vi "InitAppData.vi"(8 "error in (no error)":errorcluster, 10 "Measurement Directory":path) -> (0 "error out":errorcluster, 3 "Application Data":T1)   [LabVIEW 2019]
uses:
  Typedefs/#cluster_ApplicationData.ctl
  <vilib>/ActorFramework/Message Enqueuer/Message Enqueuer.lvclass
  Typedefs/Acquisition Thread/#cluster_AcqQueueData.ctl
  Typedefs/Acquisition Thread/#enum_AcquisitionTask.ctl
  Typedefs/Saving Thread/#cluster_SavingQueueData.ctl
  Typedefs/Saving Thread/#enum_SavingTask.ctl
  ViewerManager/ViewerManager/ViewerManager.lvclass
  C:/Program Files (x86)/National Instruments/LabVIEW 2019/vi.lib/ActorFramework/Actor/Actor.lvclass
  ViewerManager/ViewerManager Messages/UpdateMeasurementDirectory Msg/UpdateMeasurementDirectory Msg.lvclass/UpdateMeasurementDirectory Msg.ctl
  <vilib>/ActorFramework/Message Enqueuer/Message Enqueuer.lvclass/Message Enqueuer.ctl
  <vilib>/ActorFramework/Message Enqueuer/Enqueue.vi
  ViewerManager/ViewerManager Messages/UpdateMeasurementDirectory Msg/UpdateMeasurementDirectory Msg.lvclass
  C:/Program Files (x86)/National Instruments/LabVIEW 2019/vi.lib/ActorFramework/Message/Message.lvclass
  <vilib>/Utility/LVClass/Get LV Class Name.vi
  <resource>/AFDebug/Generate Trace for Message.vi
  <vilib>/ActorFramework/Message Priority Queue/Priority Enqueue.vi
  <vilib>/ActorFramework/Actor/Actor.lvclass
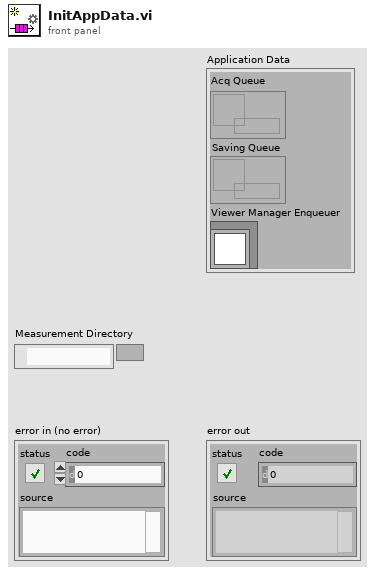
[diagram p1: front panel]
types:
  T1 = typedef "#cluster_ApplicationData.ctl" = cluster{"Acq Queue":refnum<queue>, "Saving Queue":refnum<queue>, "Viewer Manager Enqueuer":refnum<class "Message Enqueuer.lvclass">}
  T2 = typedef "#cluster_SavingQueueData.ctl" = cluster{"Task":T3, "Data":variant}
  T3 = typedef "#enum_SavingTask.ctl" = enum16{"Set directory", "Save", "Stop", "Close"}
  T4 = typedef "#cluster_AcqQueueData.ctl" = cluster{"Task":T5, "Data":variant}
  T5 = typedef "#enum_AcquisitionTask.ctl" = enum16{"Init", "Start", "Finish", "Close"}
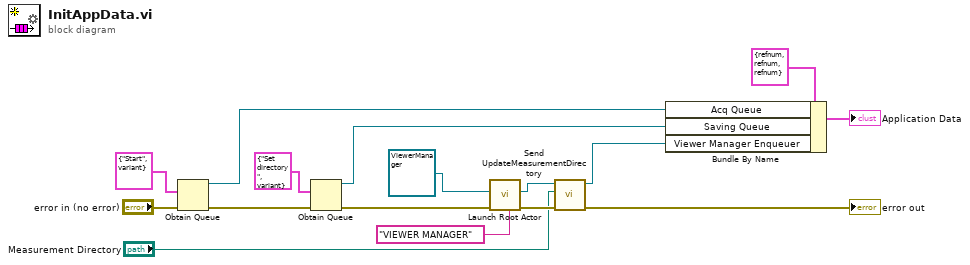
[diagram p0: block diagram]
diagram:
  n1 = Obtain Queue(element data type=T4 {"Task"=enum."Start", "Data"=variant} ("Acq Data"), error in (no error)="error in (no error)") -> (queue out=w12:refnum<queue>, error out=w15:errorcluster)  [unwired: 3 in, 1 out]
  n2 = Obtain Queue(element data type=T2 {"Task"=enum."Set directory", "Data"=variant} ("Saving Data"), error in (no error)=w15) -> (queue out=w11:refnum<queue>, error out=w7:errorcluster)  [unwired: 3 in, 1 out]
  n3 = call <vilib>:"Launch Root Actor.vi"("Debug Alias"="VIEWER MANAGER", "error in (no error)"=w7, "Actor"=refnum<class "ViewerManager.lvclass"> refnum ("ViewerManager.lvlib:ViewerManager.lvclass")) -> ("error out"=w5:errorcluster, "Actor's Enqueuer"=w4:refnum<class "Message Enqueuer.lvclass">)  [unwired: 7 in]
  n4 = call "Send UpdateMeasurementDirectory.vi"("error in (no error)"=w5, "Measurement Directory"="Measurement Directory", "Message Enqueuer"=w4) -> ("error out"=→"error out":errorcluster, "Message Enqueuer out"=w3:refnum<class "Message Enqueuer.lvclass">)  [unwired: 7 in]
  n5 = Bundle By Name(cluster=T1 {"Acq Queue"=refnum, "Saving Queue"=refnum, "Viewer Manager Enqueuer"=refnum} ("App Data"), "Acq Queue"=w12, "Saving Queue"=w11, "Viewer Manager Enqueuer"=w3) -> (→"Application Data":T1)
